vi "generate_triangle_voltages.vi"(5 "xy view?":bool, 7 "focus mode?":bool, 8 "derived values":T1, 9 "scan specification":T4={"x amplitude"=0, "x resolution (pixels)"=0, "x offset fly-forward (iterations)"=0, "x offset fly-back (iterations)"=0, "y resolution (nr. of lines)"=0, "y step size"=0, "iterations per pixel"=0, "number of frames"=0, "y offset (pixels)"=0, "number of y-brake lines  (before y-fly-back)"=0, "number y-brake lines (after y-fly-back)"=0, "number of y-fly-back steps"=8, "lines per z step"=0, "number of z/intensity tuples"=0, "number of repetitions (volumes or planes)"=0, "z step size derived"=0, "choose the beginning of z scan"=FALSE, "number of frames (settings)"=0, "FPGA trajectory?"=FALSE, "Pockels cell voltage (bits)"=0, "Vy min(bits)"=0, "Vz min(bits)"=0}, 10 "counter cluster in":T2, 11 "resonant trigger":bool) -> (0 "acquire?":bool, 1 "fly-back acquisition phase?":bool, 2 "counter cluster out":T2, 3 "DAC voltages":T3 {"ch6" max=4095 step=1; "ch5" max=4095 step=1; "ch4" max=4095 step=1; "ch3" max=4095 step=1; "ch2" max=4095 step=1; "ch1" max=4095 step=1; "ch0" max=4095 step=1}, 4 "calculate COM at the end of volume?":bool)   [LabVIEW 2010]
uses:
  scan_specification_cluster.ctl
  common_typedefs/DAC_voltage_cluster.ctl
  counter_cluster.ctl
  derived_values_cluster.ctl
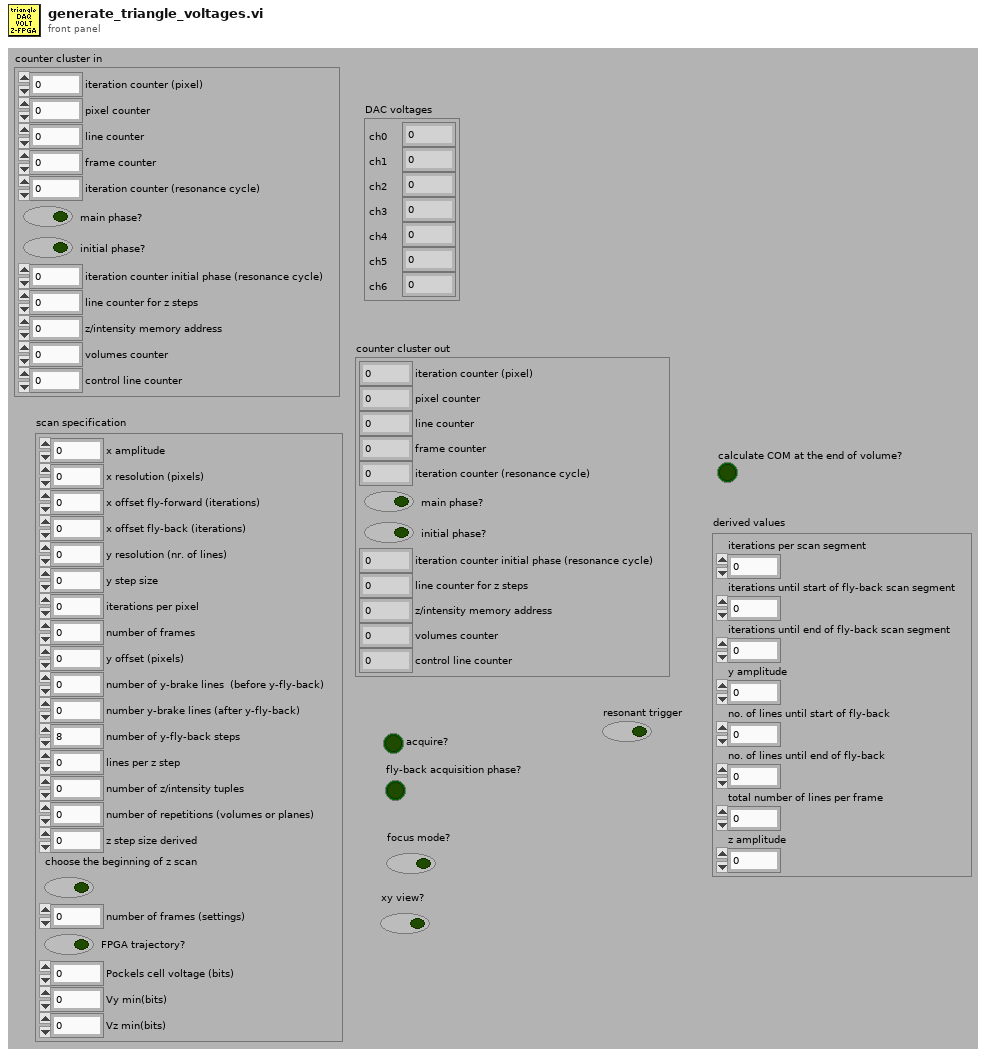
[diagram p1: front panel]
types:
  T1 = typedef "derived_values_cluster.ctl" = cluster{"iterations per scan segment":u16, "iterations until start of fly-back scan segment":u16, "iterations until end of fly-back scan segment":u16, "y amplitude":u16, "no. of lines until start of fly-back":u16, "no. of lines until end of fly-back":u16, "total number of lines per frame ":u16, "z amplitude":u16}
  T2 = typedef "counter_cluster.ctl" = cluster{"iteration counter (pixel)":u16, "pixel counter":u16, "line counter":u16, "frame counter":u16, "iteration counter (resonance cycle)":u16, "main phase?":bool, "initial phase?":bool, "iteration counter initial phase (resonance cycle)":u16, "line counter for z steps":u16, "z/intensity memory address":u32, "volumes counter":u16, "control line counter":u16}
  T3 = typedef "DAC_voltage_cluster.ctl" = cluster{"ch0":u16, "ch1":i16, "ch2":i16, "ch3":i16, "ch4":u16, "ch5":u16, "ch6":u16}
  T4 = typedef "scan_specification_cluster.ctl" = cluster{"x amplitude":u16, "x resolution (pixels)":u16, "x offset fly-forward (iterations)":u16, "x offset fly-back (iterations)":u16, "y resolution (nr. of lines)":u16, "y step size":u16, "iterations per pixel":u16, "number of frames":i32, "y offset (pixels)":u16, "number of y-brake lines  (before y-fly-back)":u16, "number y-brake lines (after y-fly-back)":u16, "number of y-fly-back steps":u16, "lines per z step":u16, "number of z/intensity tuples":u16, "number of repetitions (volumes or planes)":i32, "z step size derived":u16, "choose the beginning of z scan":bool, "number of frames (settings)":i32, "FPGA trajectory?":bool, "Pockels cell voltage (bits)":i16, "Vy min(bits)":i16, "Vz min(bits)":i16}
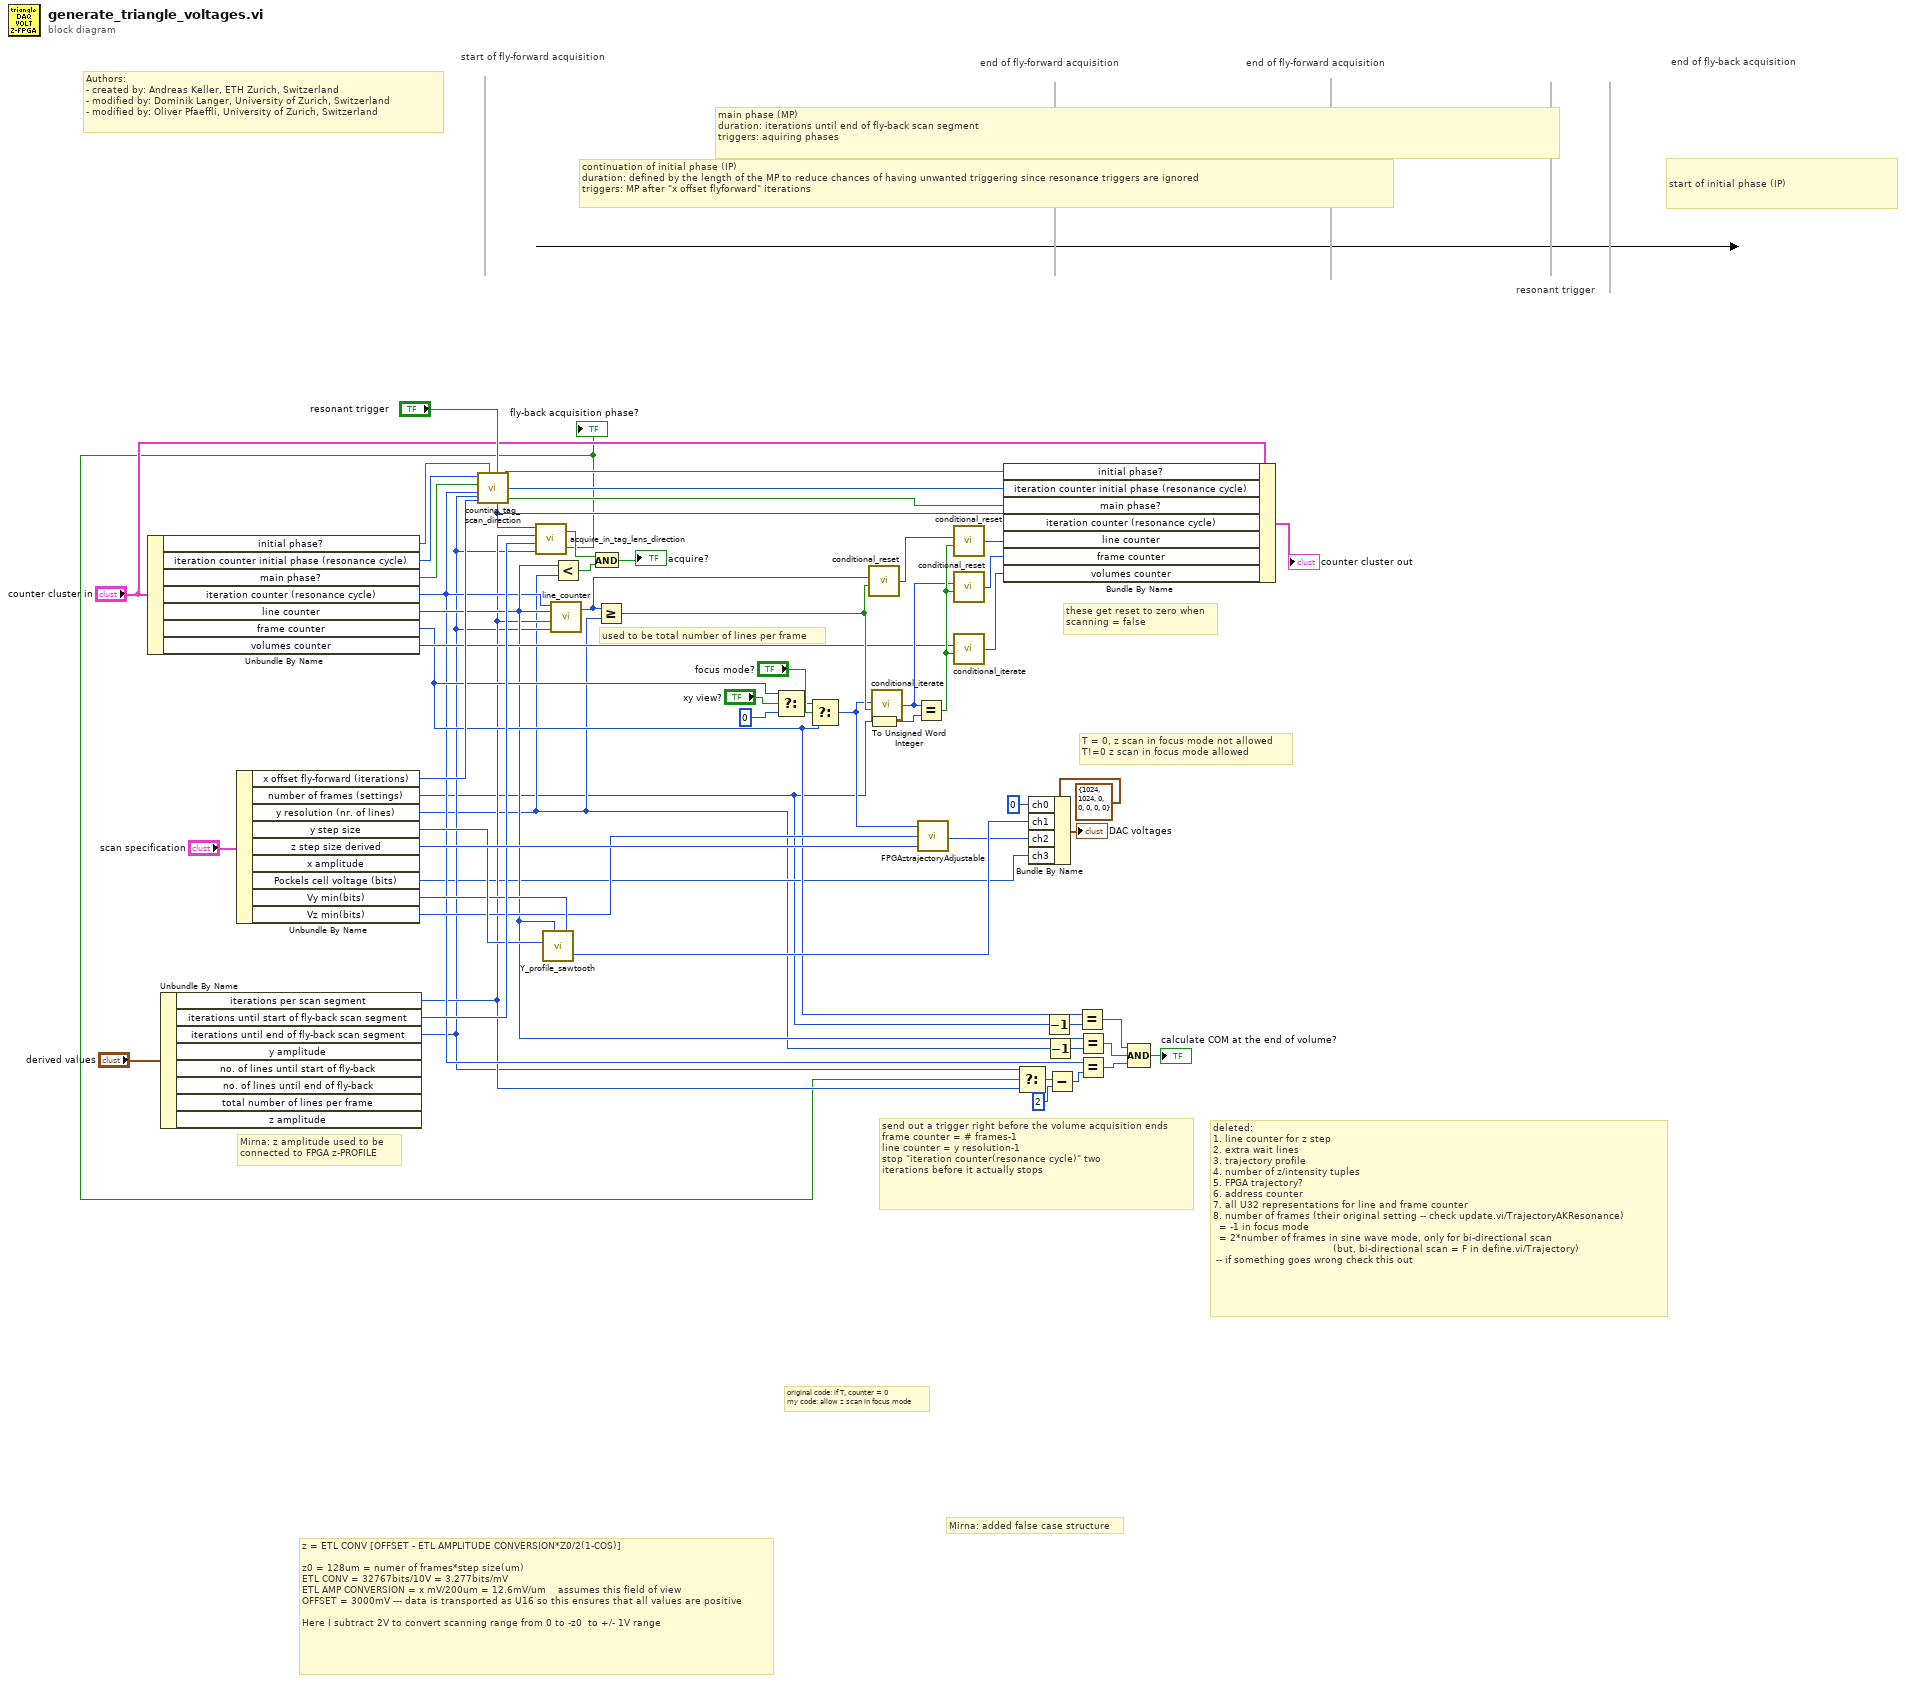
[diagram p0: block diagram]
diagram:
  # "these get reset to zero when \nscanning = false"
  # "used to be total number of lines per frame"
  # "send out a trigger right before the volume acquisition ends\nframe counter = # frames-1\nline counter = y resolution-1\nstop \"iteration counter(resonance cycle)\" two\niterations before it actually stops"
  # "Mirna: z amplitude used to be \nconnected to FPGA z-PROFILE"
  # "T = 0, z scan in focus mode not allowed\nT!=0 z scan in focus mode allowed"
  # "deleted: \n1. line counter for z step\n2. extra wait lines\n3. trajectory profile\n4. number of z/intensity tuples\n5. FPGA trajectory?\n6. address counter\n7. all U32 representations for line and frame counter\n8. number of frames (their original setting -- check update.vi/TrajectoryAKResonance)\n  = -1 in focus mode \n  = 2*number of frames in sine wave mode, only for bi-directional scan\n                                        (but, bi-directional scan = F in define.vi/Trajectory)\n -- if something goes wrong check this out"
  # "z = ETL CONV [OFFSET - ETL AMPLITUDE CONVERSION*Z0/2(1-COS)]\n\nz0 = 128um = numer of frames*step size(um)\nETL CONV = 32767bits/10V = 3.277bits/mV\nETL AMP CONVERSION = x mV/200um = 12.6mV/um    assumes this field of view\nOFFSET = 3000mV --- data is transported as U16 so this ensures that all values are positive\n\nHere I subtract 2V to convert scanning range from 0 to -z0  to +/- 1V range"
  # "original code: if T, counter = 0\nmy code: allow z scan in focus mode"
  # "Mirna: added false case structure"
  # "start of initial phase (IP)"
  # "continuation of initial phase (IP)\nduration: defined by the length of the MP to reduce chances of having unwanted triggering since resonance triggers are ignored\ntriggers: MP after \"x offset flyforward\" iterations"
  # "end of fly-back acquisition"
  # "end of fly-forward acquisition"
  # "end of fly-forward acquisition"
  # "start of fly-forward acquisition"
  # "main phase (MP)\nduration: iterations until end of fly-back scan segment\ntriggers: aquiring phases"
  # "resonant trigger"
  # "Authors: \n- created by: Andreas Keller, ETH Zurich, Switzerland\n- modified by: Dominik Langer, University of Zurich, Switzerland\n- modified by: Oliver Pfaeffli, University of Zurich, Switzerland"
  n1 = Unbundle By Name("counter cluster in") -> ("initial phase?"=w54:bool, "iteration counter initial phase (resonance cycle)"=w44:u16, "main phase?"=w51:bool, "iteration counter (resonance cycle)"=w16:u16, "line counter"=w19:u16, "frame counter"=w25:u16, "volumes counter"=w26:u16)
  n2 = Unbundle By Name("derived values") -> ("iterations per scan segment"=w15:u16, "iterations until start of fly-back scan segment"=w43:u16, "iterations until end of fly-back scan segment"=w14:u16)  [unwired: 5 out]
  n3 = Unbundle By Name("scan specification") -> ("x offset fly-forward (iterations)"=w42:u16, "number of frames (settings)"=w1:i32, "y resolution (nr. of lines)"=w3:u16, "y step size"=w40:u16, "z step size derived"=w48:u16, "Pockels cell voltage (bits)"=w4:i16, "Vy min(bits)"=w28:i16, "Vz min(bits)"=w27:i16)  [unwired: 1 out]
  n4 = call "counting_tag_scan_direction.vi"("resonant trigger"="resonant trigger", "initial phase?"=w54, "iteration counter initial phase (resonance cycle)"=w44, "main phase?"=w51, "iterations until end of fly-back scan segment"=w14, "iteration counter (resonance cycle)"=w16, "x offset fly-forward (iterations)"=w42) -> ("initial phase? OUT"=w46:bool, "iteration counter initial phase (resonance cycle) out"=w45:u16, "main phase? OUT"=w41:bool, "iteration counter (resonance cycle) out"=w39:u16)
  n5 = call "acquire_in_tag_lens_direction.vi"("iterations until end of fly-back scan segment"=w14, "iterations until start of fly-back scan segment"=w43, "iterations per scan segment"=w15, "iteration counter (resonance cycle) out"=w39) -> ("flyback phase?"=w2:bool, "acquire during flyforward or flyback phase?"=w55:bool)
  "fly-back acquisition phase?" <- w2
  n6 = call "Y_profile_sawtooth.vi"("Vy min(bits)"=w28, "line counter"=w19, "y step size"=w40) -> ("y signal"=w50:i16)  [unwired: 4 in]
  n7 = call "line_counter.vi"("iterations until end of fly-back scan segment"=w14, "iterations per scan segment"=w15, "line counter in"=w19, "iteration counter (resonance cycle)"=w16) -> ("line counter out"=w34:u16)  [unwired: 1 out]
  n8 = Less?(x=w19, y=w3) -> (x < y?=w10:bool)
  n9 = And(x=w55, y=w10) -> (x .and. y?=→"acquire?":bool)
  n10 = Greater Or Equal?(x=w34, y=w3) -> (x >= y?=w35:bool)
  n11 = Select(t=w25, s="xy view?", f=u16 0) -> (s? t:f=w29:u16)
  n12 = Select(t=w29, s="focus mode?", f=w25) -> (s? t:f=w5:u16)
  n13 = call "conditional_reset.vi"("reset?"=w35, "number in"=w34) -> ("number out"=w37:u16)  [unwired: 4 in]
  n14 = To Unsigned Word Integer(number=w1) -> (unsigned 16bit integer=w6:u16)
  n15 = call "conditional_iterate.vi"("iterate?"=w35, "number in"=w5) -> ("number out"=w33:u16)  [unwired: 4 in]
  n16 = Equal?(x=w33, y=w6) -> (x = y?=w38:bool)
  n17 = call "FPGAztrajectoryAdjustable.vi"("z step size derived"=w48, "Vz min (bits)"=w27, "z/intensity memory address"=w5) -> ("Z trajectory"=w49:i16)
  n18 = call "conditional_reset.vi"("reset?"=w38, "number in"=w37) -> ("number out"=w52:u16)  [unwired: 4 in]
  n19 = call "conditional_reset.vi"("reset?"=w38, "number in"=w33) -> ("number out"=w36:u16)  [unwired: 4 in]
  n20 = call "conditional_iterate.vi"("iterate?"=w38, "number in"=w26) -> ("number out"=w53:u16)  [unwired: 4 in]
  n21 = Bundle By Name(cluster="counter cluster in", "initial phase?"=w46, "iteration counter initial phase (resonance cycle)"=w45, "main phase?"=w41, "iteration counter (resonance cycle)"=w39, "line counter"=w52, "frame counter"=w36, "volumes counter"=w53) -> (→"counter cluster out":T2)
  n22 = Select(t=w14, s=w2, f=w15) -> (s? t:f=w13:u16)
  n23 = Bundle By Name(cluster=T3 {"ch0"=1024, "ch1"=1024, "ch2"=0, "ch3"=0, "ch4"=0, "ch5"=0, "ch6"=0} ("DAC voltage"), "ch0"=u16 0, "ch1"=w50, "ch2"=w49, "ch3"=w4) -> (→"DAC voltages":T3)
  n24 = Decrement(x=w1) -> (x-1=w24:i32)
  n25 = Decrement(x=w3) -> (x-1=w20:u16)
  n26 = Subtract(x=w13, y=u16 2) -> (x-y=w11:u16)
  n27 = Equal?(x=w25, y=w24) -> (x = y?=w23:bool)
  n28 = Equal?(x=w19, y=w20) -> (x = y?=w18:bool)
  n29 = Equal?(x=w16, y=w11) -> (x = y?=w17:bool)
  n30 = Compound Arithmetic op=AND(w23, w18, w17) -> (→"calculate COM at the end of volume?":bool)
